vi "FED.vi"(0 "System no.":i32=1 min=1 max=4 step=1, 2 "Axis to set":string[](array[string]), 3 "Parameter":i32[](array[numeric]), 5 "error in":errorcluster, 6 "Edge ID":i32[](array[numeric])) -> (19 "error out":errorcluster)   [LabVIEW 2020]
doc: "Moves given axis to a given signal edge. If multiple axes are to command, they are moved synchronously. This command does not change the reference state of the axis and does not set a certain position value. Valid Parameter values depend on EdgeID:\nEdgeID 1: negative limit switch, Parameter value is 0 when the default setting should be used (e.g. from pistages.dat), 1 when active high, -1 when active low\nEdgeID 2: positive limit switch, Parameter value is 0 when the default setting should be used (e.g. from pistages.dat), 1 when active high, -1 when active low\nEdgeID 3: reference switch, Parameter value is 0 when the default setting should be used (e.g. from pistages.dat), 1 when active high, -1 when active low\nEdgeID 4: autofind AxisIn (is one input line of the motion chip carrying an external sensor signal which changes its state at a certain position), Parameter value gives the signal state to the left of the edge (high or low) \nEdgeID 5: find arbitrary edge (i.e. change of the state of the AxisIn signal), Parameter value gives the direction of motion: 1=positive, -1= negative\n\nC-843: EdgeID can be 1 to 3. Parameter value can be -1, 0 or 1, depending on EdgeID. The firmware detects the presence or absence of reference switch and limit switches using controller parameters (ID 0x14 for reference switch; ID 0x32 for limit switches). According to the values of those parameters, the controller enables or disables FED motions to the appropriate signal edges. Adapt the parameter values to your hardware using SPA.\n\nC-867,C-877,C-884, E-861, E-871, E-873, E-874, Mercury_GCS: EdgeID can be 1 to 3. Parameter value must be 0. The firmware detects the presence or absence of reference switch and limit switches using controller parameters (ID 0x14 for reference switch; ID 0x32 for limit switches). See user manual for details and specialities. According to the values of those parameters, the controller enables or disables FED motions to the appropriate signal edges. Adapt the parameter values to your hardware using SPA or SEP.\n\nHydra, Pollux: EdgeID can be 2 or 3. Parameter value must be 0. The firmware detects the presence or absence of reference switch and limit switches using controller parameters (ID 0x14 for reference switch; ID 0x32 for limit switches). See user manual for details and specialities. According to the values of those parameters, the controller enables or disables FED motions to the appropriate signal edges. Adapt the parameter values to your hardware using SPA (or SEP, if supported)."
panel:
  # "Moves given axis to a given signal edge. If multiple axes are to command,\nthey are moved synchronously. This command does not change the reference\nstate of the axis and does not set a certain position value."
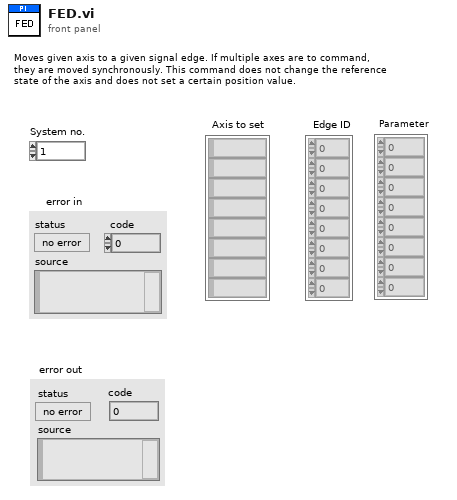
[diagram p1: front panel]
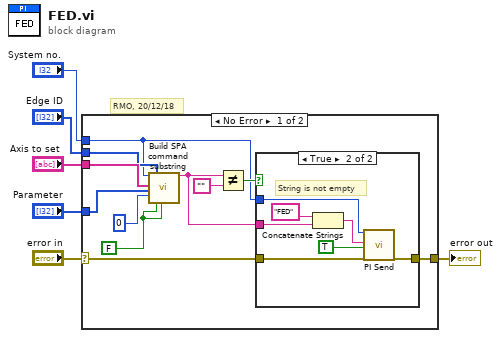
[diagram p0: block diagram]
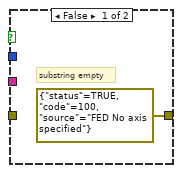
[diagram p2: hidden frame]
diagram:
  # "RMO, 20/12/18"
  n1 = case shown="No Error" "error in" {
    selector: "error in" -> [w7 w26]
    tunnel: [w17 w26] -> w6
    tunnel: "Parameter" -> [w14 _]
    tunnel: "System no." -> [w10 _]
    tunnel: "Axis to set" -> [w13 _]
    tunnel: "Edge ID" -> [w12 _]
    frame No Error {
      w8 = FALSE ("Parameter no. format \n(Decimal: FALSE)")
      n2 = call "Build SPA command substring.vi"("System no."=w10, "Axes to set"=w13, "Parameter values"=w14, "No. of digits"=i16 0, "Parameter number"=w12, "Parameter no. format \n(Decimal: FALSE)"=w8, "Parameter format \n(Num.: FALSE)"=w8) -> ("SPA command substring"=w15:string)  [unwired: 3 in, 9 out]
      n3 = Not Equal?(x=w15, y="") -> (x != y?=w11:bool)
      n4 = case shown="True" w11 {
        tunnel: w15 -> [_ w24]
        tunnel: [errorcluster {"status"=TRUE, "code"=100, "source"="FED No axis specified"} ("error out") w19] -> w17
        tunnel: w7 -> [_ w21]
        tunnel: w10 -> [_ w20]
        frame False {
          # "substring empty"
        }
        frame True {
          # "String is not empty"
          n5 = Concatenate Strings("FED", w24) -> (w22:string)
          n6 = call "PI Send.vi"("System no."=w20, "String to send"=w22, "Attach termination char.?"=TRUE ("Attach Linefeed?"), "error in"=w21) -> ("error out"=w19:errorcluster)  [unwired: 2 in, 13 out]
        }
      }
    }
    frame Error {
    }
  }
  "error out" <- w6
